vi "Extract Data Bundle.vi"(9 "IP section 4":u8, 11 "Folder Path":path) -> (3 "Data_Bundle":T1)   [LabVIEW 2013]
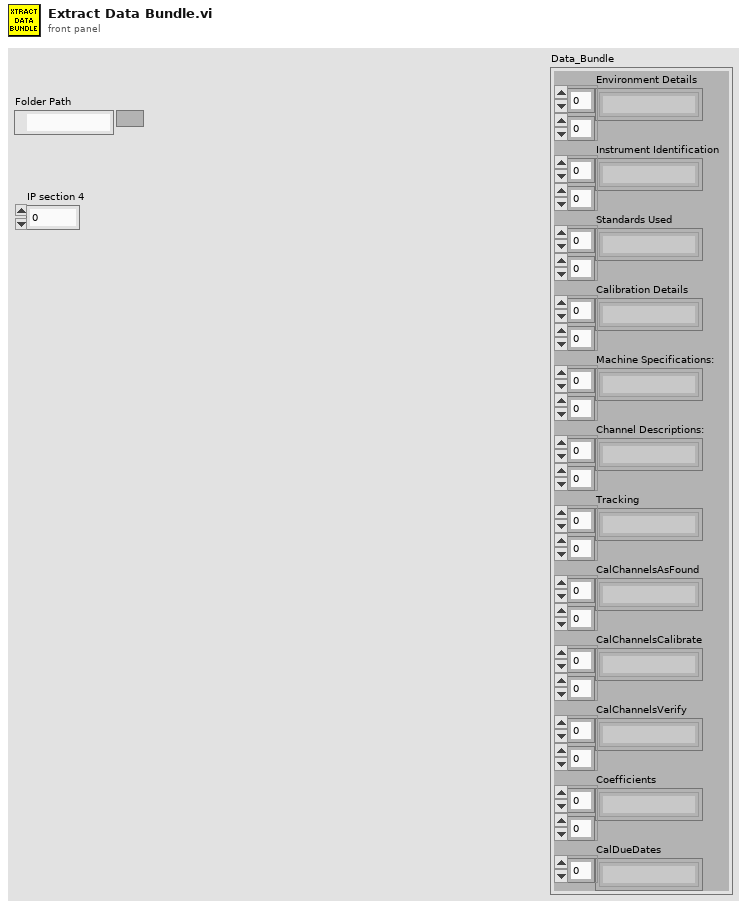
[diagram p1: front panel]
types:
  T1 = cluster{"Environment Details":string[][], "Instrument Identification":string[][], "Standards Used":string[][], "Calibration Details":string[][], "Machine Specifications:":string[][], "Channel Descriptions:":string[][], "Tracking":string[][], "CalChannelsAsFound":string[][], "CalChannelsCalibrate":string[][], "CalChannelsVerify":string[][], "Coefficients":string[][], "CalDueDates":string[]}
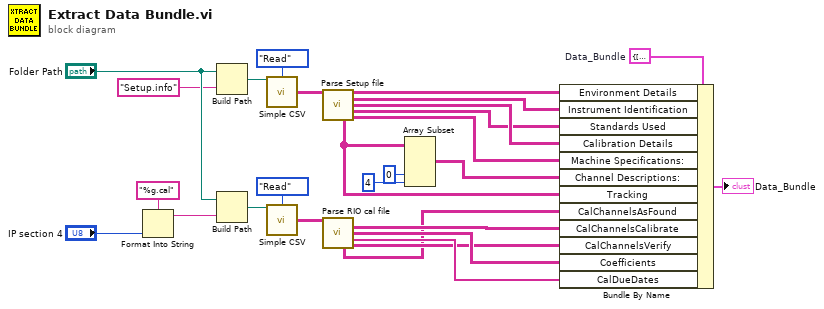
[diagram p0: block diagram]
diagram:
  w16 = T1 {"Environment Details"=[["TI Automotive"], ["Caro Test Center"], ["628 Columbia St."], ["Caro, MI 48723"], [""], [""], [""]], "Instrument Identification"=[], "Standards Used"=[], "Calibration Details"=[], "Machine Specifications:"=[], "Channel Descriptions:"=[], "Tracking"=[], "CalChannelsAsFound"=[], "CalChannelsCalibrate"=[], "CalChannelsVerify"=[], "Coefficients"=[], "CalDueDates"=[]}  # Data_Bundle
  n1 = Format Into String(format string="%g.cal", "IP section 4") -> (resulting string=w18:string)  [unwired: 2 in, 1 out]
  n2 = Build Path(base path="Folder Path", name or relative path="Setup.info") -> (appended path=w27:path)
  n3 = Build Path(base path="Folder Path", name or relative path=w18) -> (appended path=w21:path)
  n4 = call "Simple CSV.vi"("Filepath In"=w27, "Mode"=enum16{"Read", "Write"}."Read") -> ("Data Out"=w25:string[][])  [unwired: 11 in, 2 out]
  n5 = call "Simple CSV.vi"("Filepath In"=w21, "Mode"=enum16{"Read", "Write"}."Read") -> ("Data Out"=w22:string[][])  [unwired: 11 in, 2 out]
  n6 = call "Parse Setup file.vi"("Data In"=w25) -> ("Environment Details"=w15:string[][], "Instrument Identification"=w14:string[][], "Calibration Details"=w13:string[][], "Standards Used"=w12:string[][], "Channel Descriptions w/ Tracking"=w10:string[][], "Machine Specifications"=w11:string[][])  [unwired: 8 in, 1 out]
  n7 = call "Parse RIO cal file.vi"("Data In"=w22) -> ("Cal Data"=w6:string[][], "Coefficients"=w5:string[][], "Cal Dates"=w4:string[], "As Found Data"=w1:string[][], "Verify Data"=w3:string[][])  [unwired: 9 in, 1 out]
  n8 = Array Subset(array=w10, index (col)=0 ("index"), length (col)=4 ("length")) -> (w7:string[][])  [unwired: 2 in]
  n9 = Bundle By Name(cluster=w16, "Environment Details"=w15, "Instrument Identification"=w14, "Standards Used"=w12, "Calibration Details"=w13, "Machine Specifications:"=w11, "Channel Descriptions:"=w7, "Tracking"=w10, "CalChannelsAsFound"=w1, "CalChannelsCalibrate"=w6, "CalChannelsVerify"=w3, "Coefficients"=w5, "CalDueDates"=w4) -> (→"Data_Bundle":T1)
